vi "ListDevicesAfterDiscovery.vi"(11 "SCDs":refnum<class "GenericDevice.lvclass">[](array[class])) -> (3 "List of devices":string)   [LabVIEW 2023, in "DeviceManager.lvlib"]
uses:
  DeviceManager.lvlib
  Classes/GenericDevice/GenericDevice.lvclass
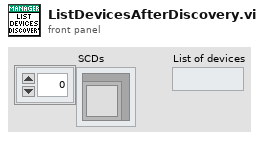
[diagram p1: front panel]
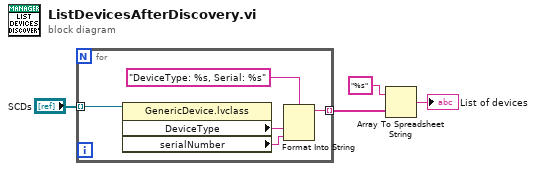
[diagram p0: block diagram]
diagram:
  n1 = for {
    tunnel: "SCDs" -> [w9] mode=indexing
    tunnel: [w5] -> w3 mode=indexing
    n2 = property class="GenericDevice.lvclass"(reference=w9) -> ("DeviceType"=w7:string, "serialNumber"=w6:string)  [unwired: 1 in, 2 out]
    n3 = Format Into String(format string="DeviceType: %s, Serial: %s", w7, w6) -> (resulting string=w5:string)  [unwired: 2 in, 1 out]
  }
  n4 = Array To Spreadsheet String(array=w3, 3:"%s" ("format string")) -> (spreadsheet string=→"List of devices":string)  [unwired: 1 in]
